vi "Write BG_level.vi"(8 "error in (no error)":errorcluster, 10 "BG_level":i32=-1, 11 "Avantes_bunch in":refnum<class "Avantes_bunch.lvclass">) -> (0 "error out":errorcluster, 3 "Avantes_bunch out":refnum<class "Avantes_bunch.lvclass">)   [LabVIEW 2020, in "Avantes_bunch.lvclass"]
uses:
  Avantes_bunch.lvclass
  Avantes_bunch.lvclass/Avantes_bunch.ctl
  Detector.lvclass
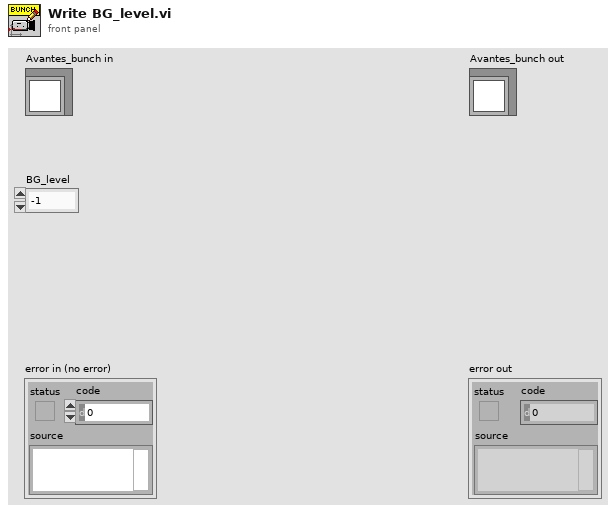
[diagram p1: front panel]
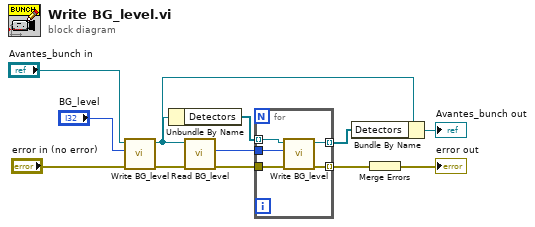
[diagram p0: block diagram]
diagram:
  n1 = call-parent "Write BG_level.vi"("error in (no error)"="error in (no error)", "BG_level"="BG_level", "Detector in"="Avantes_bunch in") -> ("error out"=w8:errorcluster, "Detector out"=w4:refnum<class "Avantes_bunch.lvclass">)  [unwired: 7 in]
  n2 = Unbundle By Name(w4) -> ("Detectors"=w9:refnum<class "Detector.lvclass">[])
  n3 = call-dynamic "Read BG_level.vi"("error in (no error)"=w8, "Detector in"=w4) -> ("error out"=w6:errorcluster, "BG_level"=w7:i32)  [unwired: 7 in, 1 out]
  n4 = for {
    tunnel: w9 -> [w16] mode=indexing
    tunnel: w7 -> [w17]
    tunnel: [w15] -> w3 mode=indexing
    tunnel: [w14] -> w5 mode=indexing
    tunnel: w6 -> [w13]
    n5 = call-dynamic "Write BG_level.vi"("error in (no error)"=w13, "BG_level"=w17, "Detector in"=w16) -> ("error out"=w14:errorcluster, "Detector out"=w15:refnum<class "Detector.lvclass">)  [unwired: 7 in]
  }
  n6 = Bundle By Name(cluster=w4, "Detectors"=w3) -> (→"Avantes_bunch out":refnum<class "Avantes_bunch.lvclass">)
  n7 = Merge Errors(w5) -> (→"error out":errorcluster)
